vi "MTS_SetGraphScales.vi"(8 "error in (no error)":errorcluster, 10 "Image Measurent Parameters":T1, 11 "Image":refnum<vi>) -> (0 "error out":errorcluster)   [LabVIEW 2013]
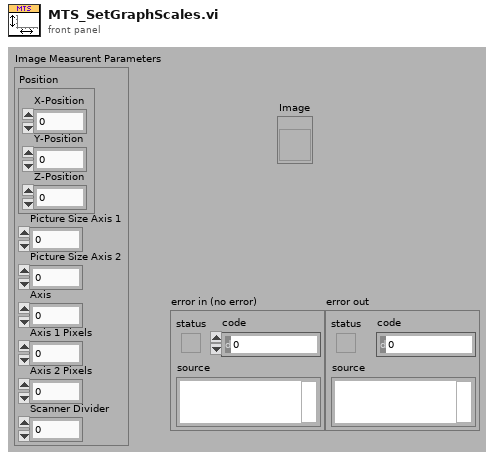
[diagram p1: front panel]
types:
  T1 = cluster{"Position":cluster{"X-Position":dbl, "Y-Position":dbl, "Z-Position":dbl}, "Picture Size Axis 1":dbl, "Picture Size Axis 2":dbl, "Axis":i32, "Axis 1 Pixels":u16, "Axis 2 Pixels":u16, "Scanner Divider":i32}
  T2 = cluster{"X-Position":dbl, "Y-Position":dbl, "Z-Position":dbl}
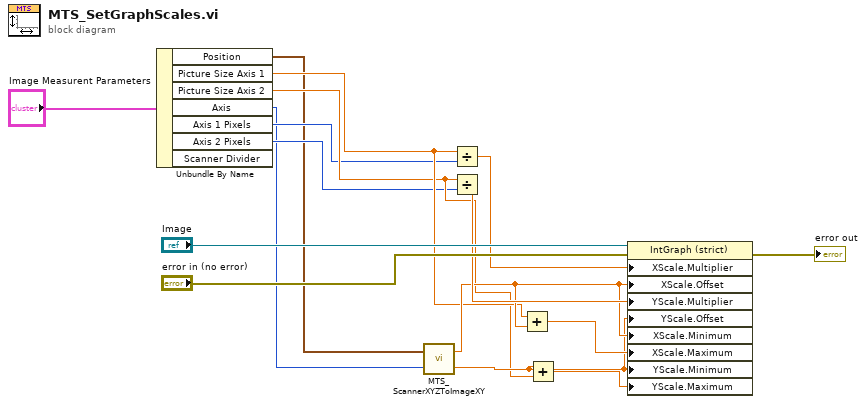
[diagram p0: block diagram]
diagram:
  n1 = Unbundle By Name("Image Measurent Parameters") -> ("Position"=w1:T2, "Picture Size Axis 1"=w6:dbl, "Picture Size Axis 2"=w5:dbl, "Axis"=w2:i32, "Axis 1 Pixels"=w4:u16, "Axis 2 Pixels"=w3:u16)  [unwired: 1 out]
  n2 = call "MTS_ScannerXYZToImageXY.vi"("Axis"=w2, "Scanner XYZ"=w1) -> ("Image Y"=w9:dbl, "Image X"=w11:dbl)
  n3 = Divide(x=w6, y=w4) -> (x/y=w13:dbl)
  n4 = Divide(x=w5, y=w3) -> (x/y=w12:dbl)
  n5 = Add(x=w6, y=w11) -> (x+y=w10:dbl)
  n6 = Add(x=w9, y=w5) -> (x+y=w8:dbl)
  n7 = property on="Property Node" class="IntGraph (strict)"(reference="Image", error in="error in (no error)", "XScale.Multiplier"=w13, "XScale.Offset"=w11, "YScale.Multiplier"=w12, "YScale.Offset"=w9, "XScale.Minimum"=w11, "XScale.Maximum"=w10, "YScale.Minimum"=w9, "YScale.Maximum"=w8) -> (error out=→"error out":errorcluster)  [unwired: 1 out]
